vi "Weather Station UI.vi"() -> ()   [LabVIEW 2012]
doc: "表示气象站项目的主VI。其中包含用于温度警告系统的用户界面。每间隔半秒读取温度；发生警告时记录数据。"
panel:
  out "警告":string
  in  "下限":dbl=20.0
  in  "上限":dbl=30.0
  in  "停止按钮":bool
  out "温度历史":dbl(graph)
  # "温度范围(C)"
  # "冷\n冻"
  # "中\n暑"
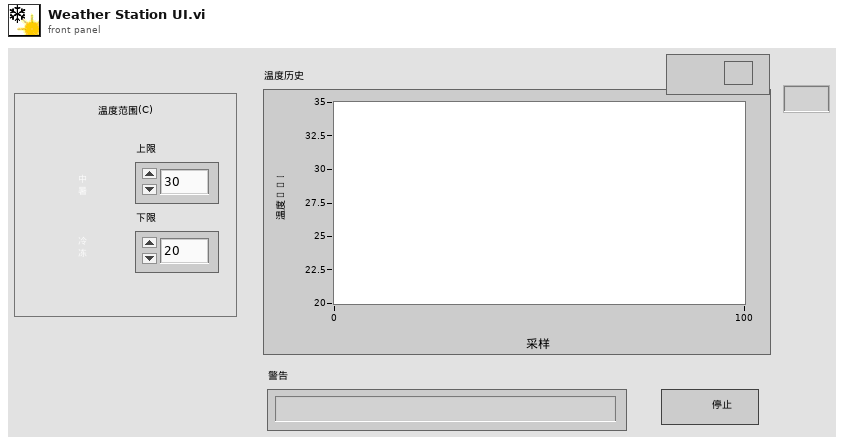
[diagram p1: front panel]
types:
  T1 = enum16{"open", "replace", "create", "open or create", "replace or create", "replace or create with confirmation"}
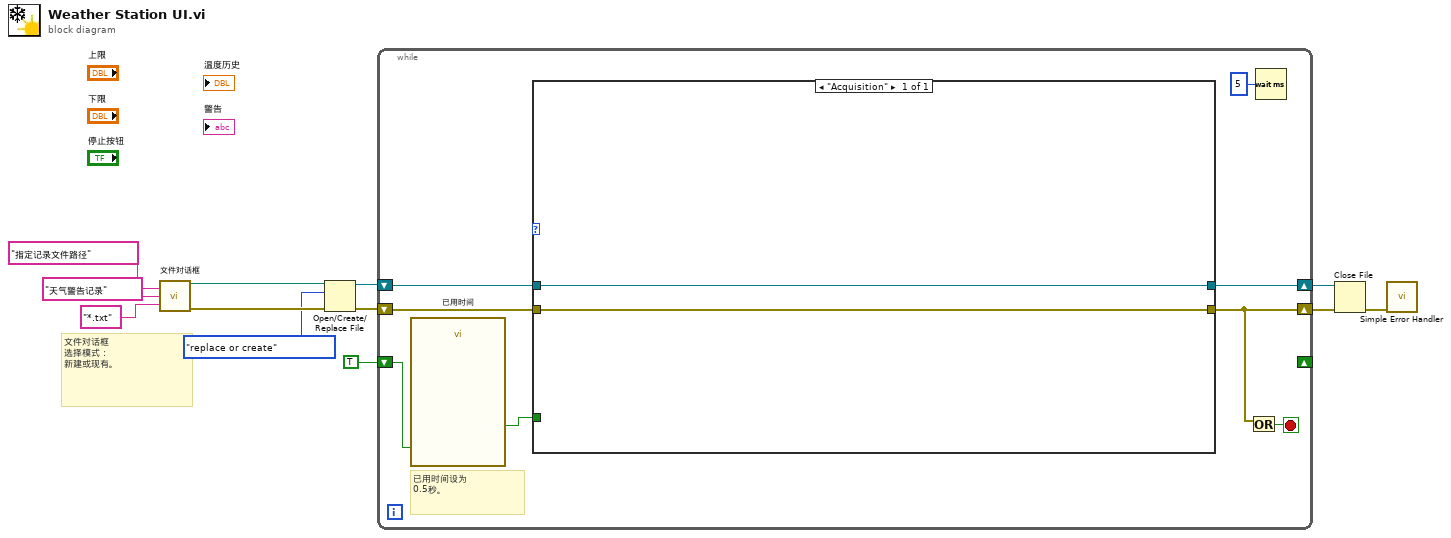
[diagram p0: block diagram]
diagram:
  # "文件对话框\n选择模式：\n新建或现有。"
  n1 = call "文件对话框"("prompt"="指定记录文件路径" ("提示"), "default name"="天气警告记录" ("默认名称"), "pattern (all files)"="*.txt" ("类型标签")) -> ("selected path"=w6:path, "error out"=w3:errorcluster)  [unwired: 9 in, 2 out]
  n2 = Open/Create/Replace File ("打开/创建/替换文件")(file path (use dialog)=w6, error in=w3, operation (0:open)=T1."replace or create" ("操作(0:open)")) -> (refnum out=w8:refnum<file>, error out=w7:errorcluster)  [unwired: 3 in, 1 out]
  n3 = while {
    shift-right: [w13] -> w12
    shift-left: w7 -> [w20]
    shift-right: [w18] -> w11
    shift-left: w8 -> [w17]
    shift-right: _ -> [_]
    shift-left: TRUE ("停止") -> [w15]
    stop <- w19 stop-if-true
    # "已用时间设为\n0.5秒。"
    n4 = call "已用时间"("Reset"=w15) -> ("Time has Elapsed"=w14:bool)  [unwired: 11 in, 7 out]
    n5 = case shown="\"采集\"" {
      selector: _ -> [_]
      tunnel: [w21] -> w13
      tunnel: w20 -> [w21]
      tunnel: [w22] -> w18
      tunnel: w17 -> [w22]
      tunnel: w14 -> [_]
      frame "Acquisition" {
      }
    }
    n6 = Or ("或")(x=w13) -> (x .or. y?=w19:bool)  [unwired: 1 in]
    n7 = Wait (ms) ("等待(ms)")(milliseconds to wait=u32 5 ("y")) -> ()  [unwired: 1 out]
  }
  n8 = Close File ("关闭文件")(refnum=w11, error in=w12) -> (error out=w10:errorcluster)  [unwired: 1 out]
  n9 = call <vilib>:"Simple Error Handler.vi"("error in (no error)"=w10) -> ()  [unwired: 4 in, 5 out]
